vi "get_non_sailpoint.vi"(1 "Waypoint queue":refnum<queue>) -> (0 "Waypoint Out":refnum<class "Waypoint.lvclass">)   [LabVIEW 2013]
doc: "Looks through the current list of waypoints and grabs the first goal point, ie the first on not marked as a sailing point."
uses:
  Classes/Waypoint/Waypoint.lvclass
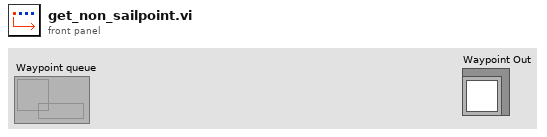
[diagram p1: front panel]
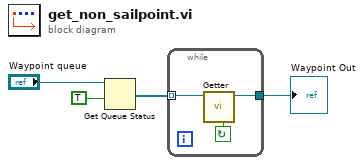
[diagram p0: block diagram]
diagram:
  n1 = Get Queue Status(queue="Waypoint queue", return elements? (F)=TRUE) -> (elements=w2:refnum<class "Waypoint.lvclass">[])  [unwired: 1 in, 7 out]
  n2 = while {
    tunnel: w2 -> [w7] mode=indexing
    tunnel: [w6] -> w1
    stop <- w5 continue-if-true
    n3 = call "Getter.vi"("Waypoint In"=w7) -> ("Waypoint Out"=w6:refnum<class "Waypoint.lvclass">, "Sailing Point?"=w5:bool)  [unwired: 5 in, 4 out]
  }
  "Waypoint Out" <- w1
